vi "Release.vi"(8 "Error In":errorcluster, 11 "Tree Data In":refnum<class "Tree Data.lvclass">) -> (0 "Error Out":errorcluster)   [LabVIEW 2016, in "Tree Data.lvclass"]
uses:
  Tree Data.lvclass
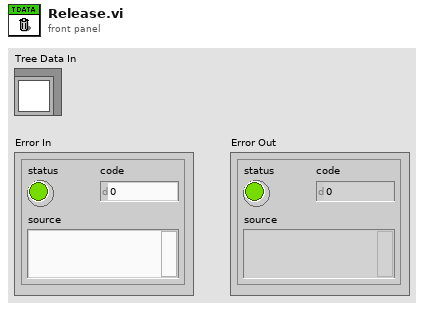
[diagram p1: front panel]
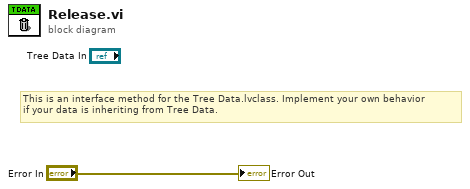
[diagram p0: block diagram]
diagram:
  # "This is an interface method for the Tree Data.lvclass. Implement your own behavior\nif your data is inheriting from Tree Data."
  "Error Out" <- "Error In"
